vi "ApplyCompensationTest.vi"() -> ()   [LabVIEW 2023]
uses:
  <vilib>/Utility/file.llb/Read Delimited Spreadsheet (DBL).vi
panel:
  out "LCR:AC Stimulus:Frequency 2":dbl format="%#_6p"
  in  "LCR:Custom Measurement Time":dbl=0.01 format="%#_6p"
  in  "LCR:Impedance Range:Impedance Range":dbl=1000000000.0 format="%#_13p"
  in  "LCR:DC Bias:Voltage Level":dbl format="%#_13g"
  in  "LCR:AC Stimulus:Voltage Amplitude":dbl=1.0 format="%#_13g"
  in  "LCR:AC Stimulus:Frequency":dbl=100000.0 format="%#_13p"
  out "OnboardCompensationData":u8[](array[numeric])
  out "Cp repeatability graph for newly performd onbaord comp and loaded comp":dbl[][](graph)
  out "LoadedCompensationData":u8[](array[numeric])
  out "error out":errorcluster
  in  "resource name":refnum<k15>="LCR_4190_C02_S08"
  # "Warning 1073364993\nNow after putting 10ms there"
  # "If measurement time is too high for 100 singlepoint measurements"
  # "Went away after wait was implemented before first measurement"
  # "-1074116981"
  # "niDCPower Measure Multiple LCR.vi<ERR>Internal Hardware Error. Contact NI support.\n\nDevice: LCR_4190_C02_S08/0\nAdditional Error Info: Captured Board: 0, Iso Captured Channel: [776], Sticky Board: [], Iso Errors Available: 1, Iso Sticky Channel: [[776]], Errors Version: 4.6.0f106, Last Completed Setup Level: 15"
  # "Wait for source done event was not implemented correctly yet."
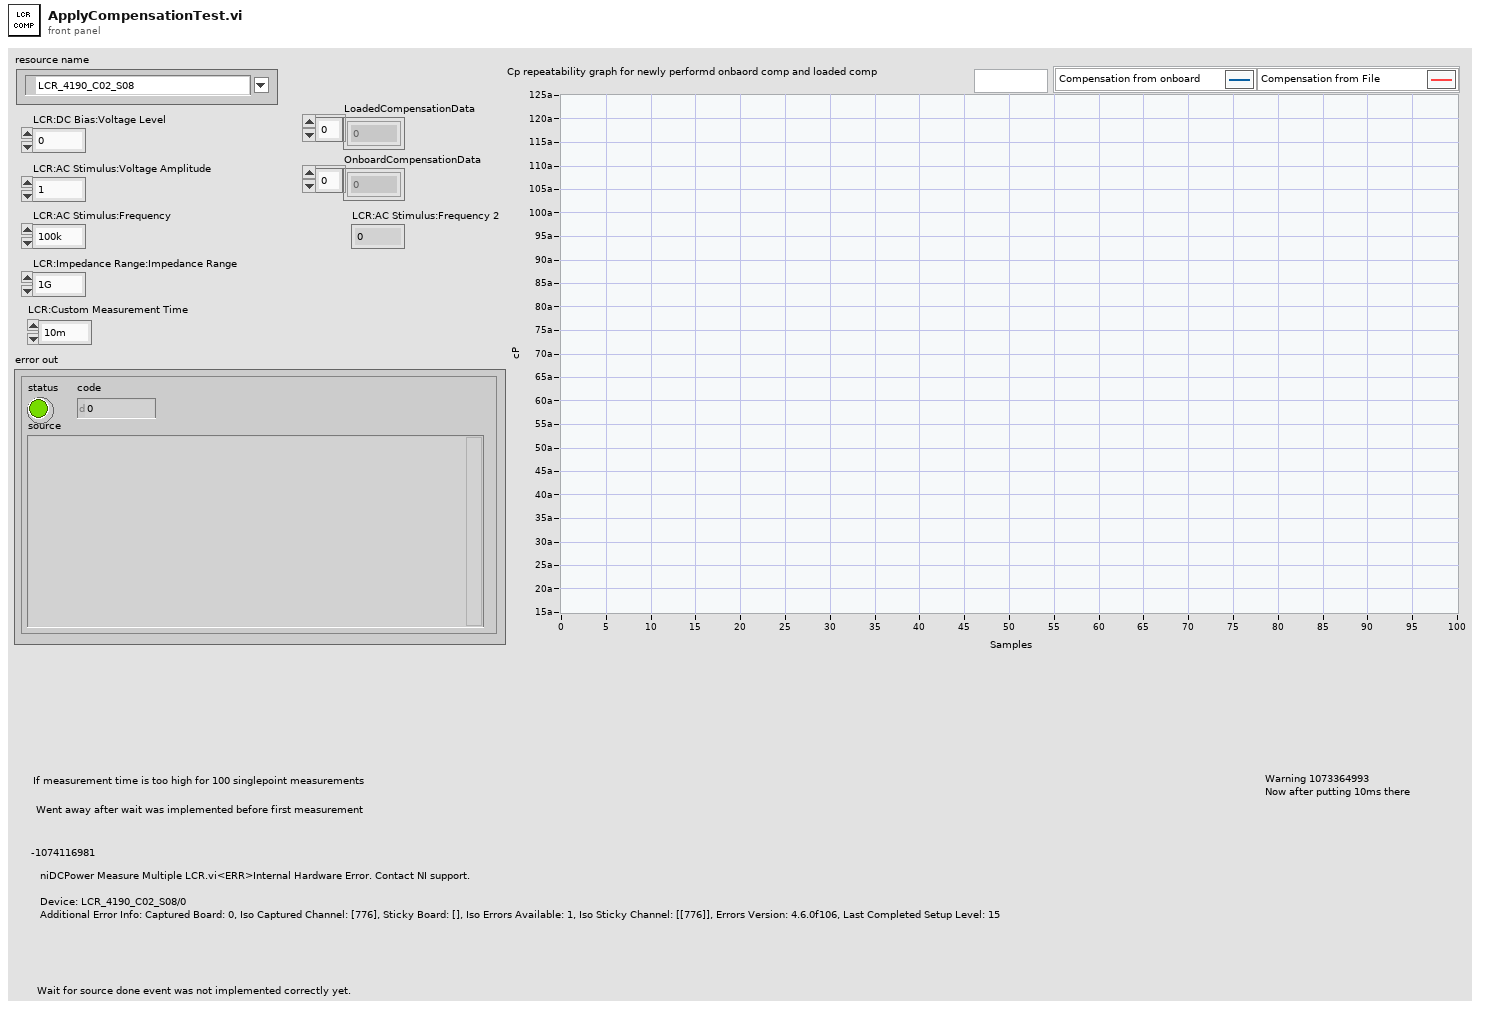
[diagram p1: front panel]
types:
  T1 = typedef "niDCPower LCR Measurement.ctl" = cluster{"V DC":dbl, "I DC":dbl, "stimulus frequency":dbl, "AC voltage":cdb, "AC current":cdb, "Z":cdb, "Z magnitude":dbl, "Z theta":dbl, "Y":cdb, "Y magnitude":dbl, "Y theta":dbl, "Ls":dbl, "Cs":dbl, "Rs":dbl, "Lp":dbl, "Cp":dbl, "Rp":dbl, "D":dbl, "Q":dbl, "measurement mode":u16, "DC in compliance":bool, "Pad 0":u8, "AC in compliance":bool, "Pad 1":u8, "unbalanced":bool, "Pad 2":u8, "Reserved 1":dbl, "Reserved 2":dbl, "Reserved 3":dbl, "Reserved 4":dbl, "Reserved 5":dbl, "Reserved 6":dbl, "Reserved 7":dbl}
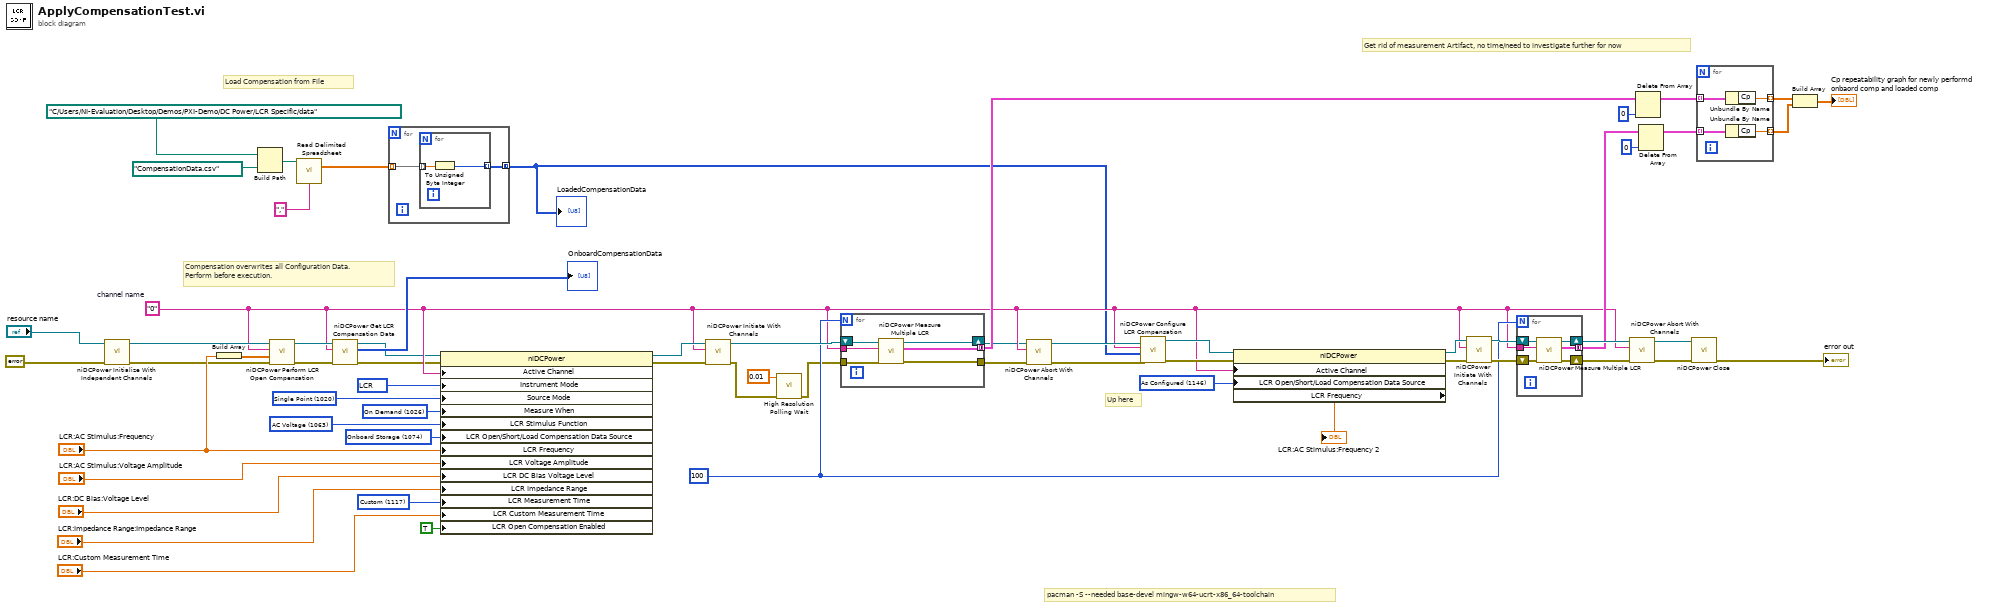
[diagram p0: block diagram]
diagram:
  w21 = 1117 items=["Short"=1071, "Medium"=1072, "Long"=1073, "Custom"=1117] ("LCR:Measurement Time")
  w29 = 1074 items=["Onboard Storage"=1074, "As Defined"=1075, "As Configured"=1146] ("LCR:Compensation:LCR Open/Short/Load Compensation Data Source")
  w1 = 1146 items=["Onboard Storage"=1074, "As Defined"=1075, "As Configured"=1146] ("LCR:Compensation:LCR Open/Short/Load Compensation Data Source")
  w35 = 1026 items=["Automatically after Source Complete"=1025, "On Demand"=1026, "On Measure Trigger"=1027] ("Measurement:Advanced:Measure When")
  w36 = 1020 items=["Single Point"=1020, "Sequence"=1021] ("Source:Source Mode")
  w53 = 1063 items=["AC Voltage"=1063, "AC Current"=1064] ("LCR:AC Stimulus:Function")
  w30 = 100 ("count (1)")
  w61 = 1062 items=["SMU PS"=1061, "LCR"=1062, "E-Load"=1154] ("LCR:Instrument Mode")
  w7 = "0"  # channel name
  # "pacman -S --needed base-devel mingw-w64-ucrt-x86_64-toolchain"
  # "Get rid of measurement Artifact, no time/need to investigate further for now"
  # "Compensation overwrites all Configuration Data.\nPerform before execution."
  # "Load Compensation from File"
  # "Up here"
  n1 = call <instrlib>:"niDCPower Initialize With Independent Channels.vi"("error in (no error)"=errorcluster {"status"=FALSE, "code"=0, "source"=""}, "resource name"="resource name") -> ("error out"=w24:errorcluster, "instrument handle out"=w25:refnum<k15>)  [unwired: 8 in]
  n2 = Build Array("LCR:AC Stimulus:Frequency") -> (w26:dbl[])
  n3 = Build Path(base path=path "C:/Users/NI-Evaluation/Desktop/Demos/PXI-Demo/DC Power/LCR Specific/data", name or relative path=path "CompensationData.csv") -> (appended path=w38:path)
  n4 = call <instrlib>:"niDCPower Perform LCR Open Compensation.vi"("error in (no error)"=w24, "additional frequencies"=w26, "channel name"=w7, "instrument handle"=w25) -> ("error out"=w9:errorcluster, "instrument handle out"=w8:refnum<k15>)  [unwired: 6 in]
  n5 = call-poly <vilib>:"Read Delimited Spreadsheet.vi"("file path (dialog if empty)"=w38, "delimiter (\\t)"="," ("delimiter (\\t)")) -> ("all rows"=w37:dbl[][])  [unwired: 8 in, 5 out]
  n6 = call <instrlib>:"niDCPower Get LCR Compensation Data.vi"("error in (no error)"=w9, "channel name"=w7, "instrument handle"=w8) -> ("error out"=w5:errorcluster, "compensation data"=→"OnboardCompensationData":u8[], "instrument handle out"=w6:refnum<k15>)  [unwired: 6 in]
  n7 = for {
    tunnel: w37 -> [w64] mode=indexing
    tunnel: [w63] -> w2 mode=concatenating
    n8 = for {
      tunnel: w64 -> [w66] mode=indexing
      tunnel: [w65] -> w63 mode=indexing
      n9 = To Unsigned Byte Integer(number=w66) -> (unsigned 8bit integer=w65:u8)
    }
  }
  "LoadedCompensationData" <- w2
  n10 = property class="niDCPower"(reference=w6, error in=w5, "Active Channel"=w7, "Instrument Mode"=w61, "Source Mode"=w36, "Measure When"=w35, "LCR Stimulus Function"=w53, "LCR Open/Short/Load Compensation Data Source"=w29, "LCR Frequency"="LCR:AC Stimulus:Frequency", "LCR Voltage Amplitude"="LCR:AC Stimulus:Voltage Amplitude", "LCR DC Bias Voltage Level"="LCR:DC Bias:Voltage Level", "LCR Impedance Range"="LCR:Impedance Range:Impedance Range", "LCR Measurement Time"=w21, "LCR Custom Measurement Time"="LCR:Custom Measurement Time", "LCR Open Compensation Enabled"=TRUE ("LCR:Compensation:Open:Enabled")) -> (reference out=w22:refnum<k15>, error out=w23:errorcluster)
  n11 = call <instrlib>:"niDCPower Initiate With Channels.vi"("error in (no error)"=w23, "channel name"=w7, "instrument handle"=w22) -> ("error out"=w12:errorcluster, "instrument handle out"=w47:refnum<k15>)  [unwired: 7 in]
  n12 = call <vilib>:"High Resolution Polling Wait.vi"("error in (no error)"=w12, "seconds to wait"=0.01) -> ("error out"=w11:errorcluster)  [unwired: 9 in]
  n13 = for {
    N: w30 -> [_]
    tunnel: w7 -> [w71]
    tunnel: [w70] -> w19 mode=concatenating
    shift-right: [w68] -> w4
    shift-left: w47 -> [w69]
    tunnel: w11 -> [w72]
    tunnel: [w67] -> w3
    n14 = call <instrlib>:"niDCPower Measure Multiple LCR.vi"("error in (no error)"=w72, "channel name"=w71, "instrument handle"=w69) -> ("error out"=w67:errorcluster, "measurements"=w70:T1[], "instrument handle out"=w68:refnum<k15>)  [unwired: 6 in]
  }
  n15 = call <instrlib>:"niDCPower Abort With Channels.vi"("error in (no error)"=w3, "channel name"=w7, "instrument handle"=w4) -> ("error out"=w48:errorcluster, "instrument handle out"=w46:refnum<k15>)  [unwired: 7 in]
  n16 = call <instrlib>:"niDCPower Configure LCR Compensation.vi"("error in (no error)"=w48, "compensation data"=w2, "channel name"=w7, "instrument handle"=w46) -> ("error out"=w45:errorcluster, "instrument handle out"=w44:refnum<k15>)  [unwired: 6 in]
  n17 = property class="niDCPower"(reference=w44, error in=w45, "Active Channel"=w7, "LCR Open/Short/Load Compensation Data Source"=w1) -> (reference out=w42:refnum<k15>, error out=w43:errorcluster, "LCR Frequency"=→"LCR:AC Stimulus:Frequency 2":dbl)
  n18 = call <instrlib>:"niDCPower Initiate With Channels.vi"("error in (no error)"=w43, "channel name"=w7, "instrument handle"=w42) -> ("error out"=w59:errorcluster, "instrument handle out"=w60:refnum<k15>)  [unwired: 7 in]
  n19 = for {
    N: w30 -> [_]
    tunnel: w7 -> [w78]
    tunnel: [w76] -> w18 mode=concatenating
    shift-right: [w77] -> w58
    shift-left: w60 -> [w73]
    shift-right: [w75] -> w57
    shift-left: w59 -> [w74]
    n20 = call <instrlib>:"niDCPower Measure Multiple LCR.vi"("error in (no error)"=w74, "channel name"=w78, "instrument handle"=w73) -> ("error out"=w75:errorcluster, "measurements"=w76:T1[], "instrument handle out"=w77:refnum<k15>)  [unwired: 6 in]
  }
  n21 = call <instrlib>:"niDCPower Abort With Channels.vi"("error in (no error)"=w57, "channel name"=w7, "instrument handle"=w58) -> ("error out"=w55:errorcluster, "instrument handle out"=w56:refnum<k15>)  [unwired: 7 in]
  n22 = Delete From Array(array=w19, index=0) -> (array with subset deleted=w14:T1[])  [unwired: 1 in, 1 out]
  n23 = Delete From Array(array=w18, index=0) -> (array with subset deleted=w17:T1[])  [unwired: 1 in, 1 out]
  n24 = call <instrlib>:"niDCPower Close.vi"("error in (no error)"=w55, "instrument handle"=w56) -> ("error out"=→"error out":errorcluster)  [unwired: 9 in]
  n25 = for {
    tunnel: w14 -> [w82] mode=indexing
    tunnel: w17 -> [w81] mode=indexing
    tunnel: [w80] -> w33 mode=indexing
    tunnel: [w79] -> w32 mode=indexing
    n26 = Unbundle By Name(w82) -> ("Cp"=w80:dbl)
    n27 = Unbundle By Name(w81) -> ("Cp"=w79:dbl)
  }
  n28 = Build Array(w33, w32) -> (→"Cp repeatability graph for newly performd onbaord comp and loaded comp":dbl[][])
